vi "Get I32 Value from HashTable.vi"(8 "error in (no error)":errorcluster caption="错误输入（无错误）", 10 "Name":string, 11 "Contstant Base 输入":refnum<class "Tag Data.lvclass"> caption="DNL_LabVIEW Object in") -> (0 "error out":errorcluster caption="错误输出", 2 "Value":i32, 3 "Contstant Base 输出":refnum<class "Tag Data.lvclass"> caption="DNL_LabVIEW Object out")   [LabVIEW 2013, in "Tag Data.lvclass"]
uses:
  Tag Data.lvclass
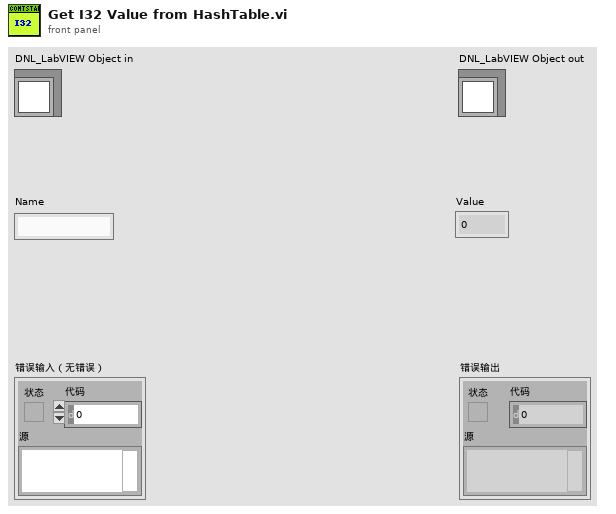
[diagram p1: front panel]
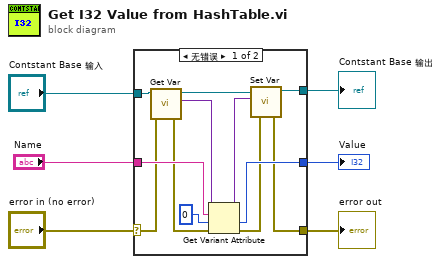
[diagram p0: block diagram]
diagram:
  n1 = case shown="无错误" "error in (no error)" {
    selector: "error in (no error)" -> [w11 w20]
    tunnel: [w8 w20] -> w5
    tunnel: [w12 w19] -> w3
    tunnel: "Contstant Base 输入" -> [w17 w19]
    tunnel: "Name" -> [w18 _]
    tunnel: [w13 _] -> w1
    frame No Error {
      n2 = call-dynamic "Get Var.vi"("error in (no error)"=w11, "Contstant Base输入"=w17) -> ("error out"=w10:errorcluster, "Var"=w15:variant, "Contstant Base输出"=w16:refnum<class "Tag Data.lvclass">)  [unwired: 7 in]
      n3 = Get Variant Attribute(Variant=w15, name=w18, default value (empty Variant)=0, error in=w10) -> (duplicate Variant=w14:variant, value=w13:i32, error out=w9:errorcluster)  [unwired: 1 out]
      n4 = call-dynamic "Set Var.vi"("error in (no error)"=w9, "Var"=w14, "Contstant Base输入"=w16) -> ("error out"=w8:errorcluster, "Contstant Base输出"=w12:refnum<class "Tag Data.lvclass">)  [unwired: 7 in]
    }
    frame Error {
    }
  }
  "error out" <- w5
  "Contstant Base 输出" <- w3
  "Value" <- w1
